vi "cursor manipulation.vi"(5 "cursor type":T1(ring), 6 "Cursor.Cursor Mode":u32, 7 "cursor position":T4(ring), 9 "graph reference in":refnum<vi>, 10 "y-array":dbl[](array[numeric]), 11 "x-array":dbl[](array[numeric])) -> (3 "reference out":refnum<vi>)   [LabVIEW 2021]
uses:
  <vilib>/Utility/miscctls.llb/LVCursorListTypeDef.ctl
panel:
  out "Cursor List Out":T2(array[cluster])
  out "Cursor List In":T3=[{"Name"="Cursor 0", "Color"=16775680, "Style"=0, "Point Style"=13, "Name Visible"=FALSE, "Allow Drag"=TRUE, "Cursor Mode"=1, "Plot"=0, "Index"=0, "Position"={"X"=99.93178733333333, "Y"=99.0278}, "X Scale"=0, "Y Scale"=0, "Watch Plots"=[], "Watch All Plots"=FALSE, "Plot Area"=0, "Label Offset"={"X"=-47.70298455485651, "Y"=-2401.3690448763255}}, {"Name"="Cursor 1", "Color"=16776960, "Style"=0, "Point Style"=13, "Name Visible"=FALSE, "Allow Drag"=TRUE, "Cursor Mode"=1, "Plot"=-1, "Index"=33, "Position"={"X"=197.3124, "Y"=196.0}, "X Scale"=0, "Y Scale"=0, "Watch Plots"=[], "Watch All Plots"=FALSE, "Plot Area"=0, "Label Offset"={"X"=24.672569516556308, "Y"=-2417.1156279151946}}]
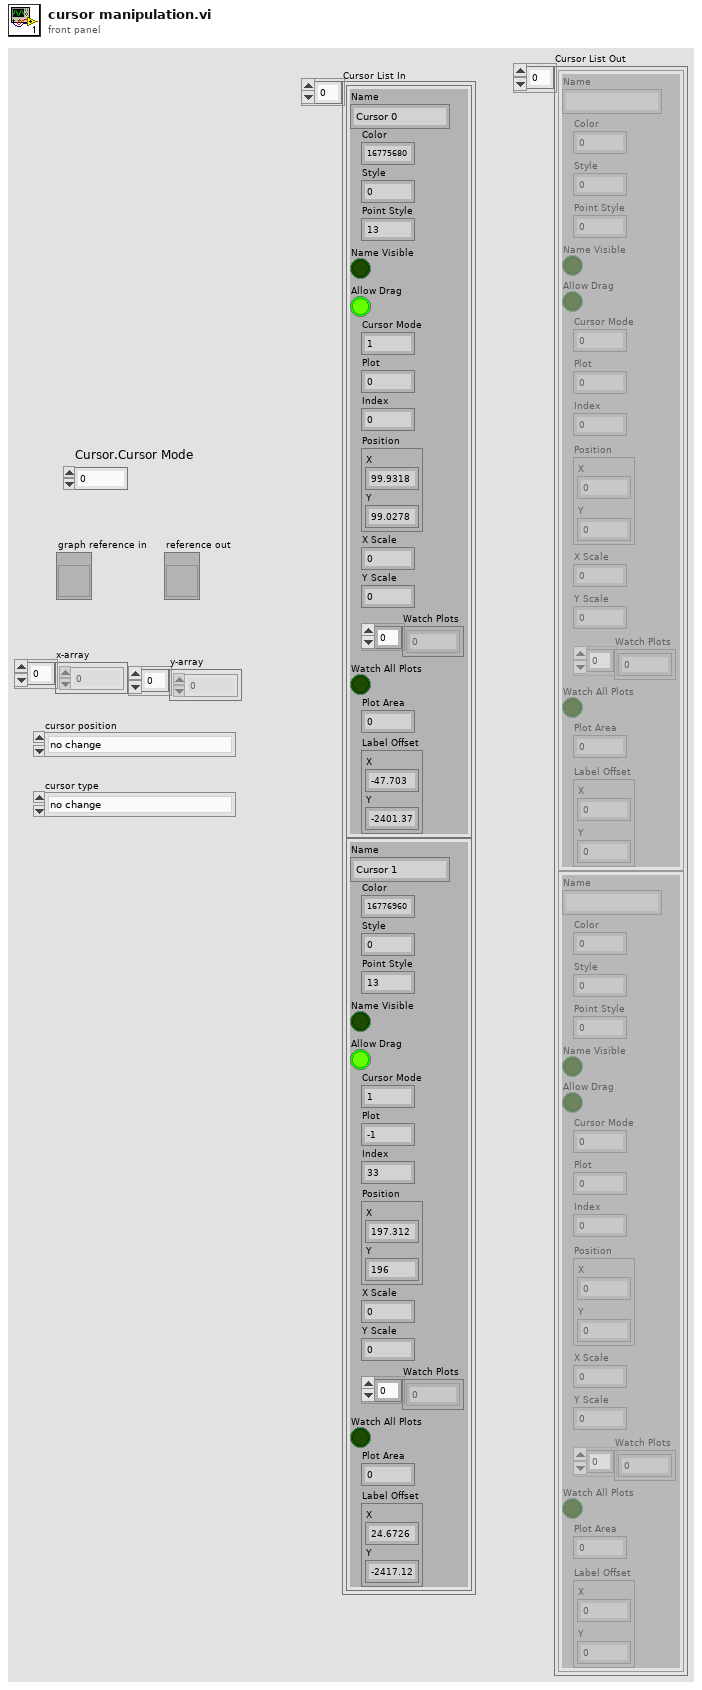
[diagram p1: front panel]
types:
  T1 = enum16{"no change", "hide cursor", "cross", "horizontal", "vertical"}
  T2 = cluster{"Name":string, "Color":u32, "Style":u8, "Point Style":u8, "Name Visible":bool, "Allow Drag":bool, "Cursor Mode":u32, "Plot":i32, "Index":i32, "Position":cluster{"X":dbl, "Y":dbl}, "X Scale":u32, "Y Scale":u32, "Watch Plots":i32[], "Watch All Plots":bool, "Plot Area":i32, "Label Offset":cluster{"X":dbl, "Y":dbl}}[]
  T3 = typedef "LVCursorListTypeDef.ctl" = cluster{"Name":string, "Color":u32, "Style":u8, "Point Style":u8, "Name Visible":bool, "Allow Drag":bool, "Cursor Mode":u32, "Plot":i32, "Index":i32, "Position":cluster{"X":dbl, "Y":dbl}, "X Scale":u32, "Y Scale":u32, "Watch Plots":i32[], "Watch All Plots":bool, "Plot Area":i32, "Label Offset":cluster{"X":dbl, "Y":dbl}}[]
  T4 = enum16{"no change", "move to data center", "move to data corner", "move to panel center", "move to panel corner"}
  T5 = cluster{"Name":string, "Color":u32, "Style":u8, "Point Style":u8, "Name Visible":bool, "Allow Drag":bool, "Cursor Mode":u32, "Plot":i32, "Index":i32, "Position":cluster{"X":dbl, "Y":dbl}, "X Scale":u32, "Y Scale":u32, "Watch Plots":i32[], "Watch All Plots":bool, "Plot Area":i32, "Label Offset":cluster{"X":dbl, "Y":dbl}}
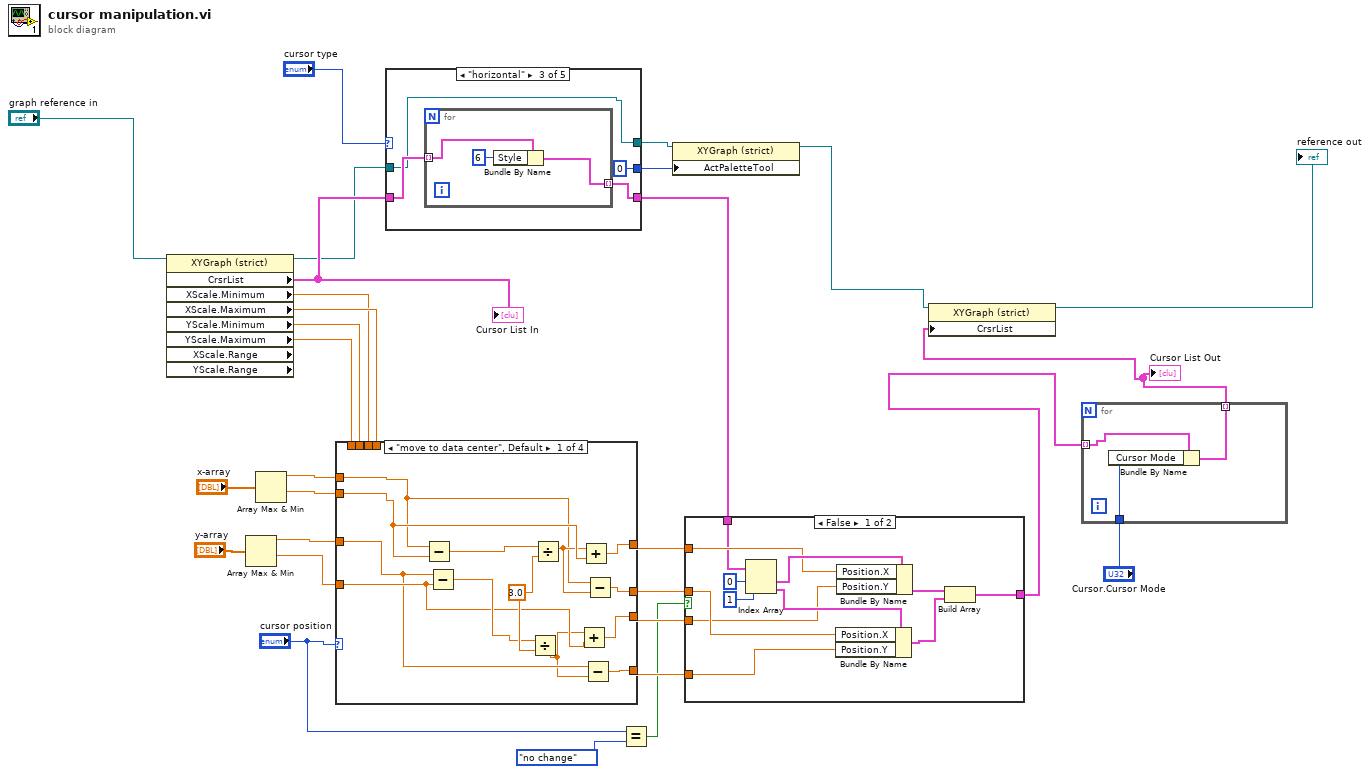
[diagram p0: block diagram]
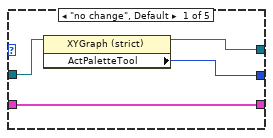
[diagram p3: hidden frame]
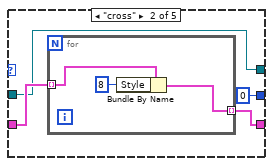
[diagram p4: hidden frame]
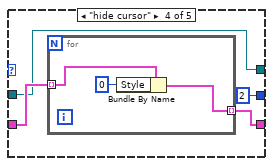
[diagram p5: hidden frame]
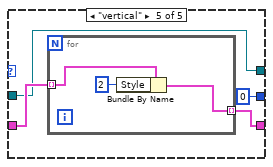
[diagram p6: hidden frame]
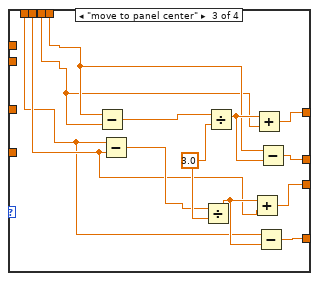
[diagram p8: hidden frame]
diagram:
  n1 = property on="Property Node" class="XYGraph (strict)" props=["CrsrList", "XScale", "Minimum", "XScale", "Maximum", "YScale", "Minimum", "YScale", "Maximum", "XScale", "Range", "YScale", "Range"](reference="graph reference in") -> (reference out=w9:refnum<vi>, "CrsrList"=w14:T3, "XScale.Minimum"=w18:dbl, "XScale.Maximum"=w19:dbl, "YScale.Minimum"=w17:dbl, "YScale.Maximum"=w16:dbl)  [unwired: 1 in, 3 out]
  "Cursor List In" <- w14
  n2 = Array Max & Min(array="y-array") -> (max value=w22:dbl, min value=w23:dbl)  [unwired: 2 out]
  n3 = Array Max & Min(array="x-array") -> (max value=w26:dbl, min value=w27:dbl)  [unwired: 2 out]
  n4 = case shown="\"move to data center\", Default" "cursor position" {
    tunnel: w27 -> [w39 w44 _ _]
    tunnel: w26 -> [w37 _ _ _]
    tunnel: [w36 w44 w52 w59] -> w25
    tunnel: [w35 w44 w51 w59] -> w24
    tunnel: w23 -> [w34 w43 _ _]
    tunnel: w22 -> [w33 _ _ _]
    tunnel: [w32 w43 w50 w58] -> w21
    tunnel: [w31 w43 w49 w58] -> w20
    tunnel: w19 -> [_ _ w48 _]
    tunnel: w18 -> [_ _ w47 w59]
    tunnel: w17 -> [_ _ w46 w58]
    tunnel: w16 -> [_ _ w45 _]
    frame "move to data center", Default {
      w41 = 3.0 ("y")
      n5 = Subtract(x=w37, y=w39) -> (x-y=w42:dbl)
      n6 = Subtract(x=w33, y=w34) -> (x-y=w40:dbl)
      n7 = Divide(x=w40, y=w41) -> (x/y=w30:dbl)
      n8 = Divide(x=w42, y=w41) -> (x/y=w38:dbl)
      n9 = Add(x=w30, y=w34) -> (x+y=w32:dbl)
      n10 = Add(x=w38, y=w39) -> (x+y=w36:dbl)
      n11 = Subtract(x=w33, y=w30) -> (x-y=w31:dbl)
      n12 = Subtract(x=w37, y=w38) -> (x-y=w35:dbl)
    }
    frame "move to data corner" {
    }
    frame "move to panel center" {
      w56 = 3.0 ("y")
      n13 = Subtract(x=w48, y=w47) -> (x-y=w57:dbl)
      n14 = Subtract(x=w45, y=w46) -> (x-y=w55:dbl)
      n15 = Divide(x=w55, y=w56) -> (x/y=w54:dbl)
      n16 = Divide(x=w57, y=w56) -> (x/y=w53:dbl)
      n17 = Add(x=w54, y=w46) -> (x+y=w50:dbl)
      n18 = Add(x=w53, y=w47) -> (x+y=w52:dbl)
      n19 = Subtract(x=w45, y=w54) -> (x-y=w49:dbl)
      n20 = Subtract(x=w48, y=w53) -> (x-y=w51:dbl)
    }
    frame "move to panel corner" {
    }
  }
  n21 = case shown="\"horizontal\"" "cursor type" {
    tunnel: w14 -> [w63 w67 w74 w81 w88]
    tunnel: [w63 w66 w73 w80 w87] -> w13
    tunnel: w9 -> [w62 w65 w72 w79 w86]
    tunnel: [w61 w65 w72 w79 w86] -> w8
    tunnel: [w60 0 ("ActPaletteTool") 0 ("ActPaletteTool") 2 ("ActPaletteTool") 0 ("ActPaletteTool")] -> w7
    frame "no change", Default {
      n22 = property class="XYGraph (strict)"(reference=w62) -> (reference out=w61:refnum<vi>, "ActPaletteTool"=w60:i32)  [unwired: 1 in, 1 out]
    }
    frame "cross" {
      n23 = for {
        tunnel: w67 -> [w70] mode=indexing
        tunnel: [w68] -> w66 mode=indexing
        n24 = Bundle By Name(cluster=w70, "Style"=u8 8) -> (w68:T5)
      }
    }
    frame "horizontal" {
      n25 = for {
        tunnel: w74 -> [w77] mode=indexing
        tunnel: [w75] -> w73 mode=indexing
        n26 = Bundle By Name(cluster=w77, "Style"=u8 6) -> (w75:T5)
      }
    }
    frame "hide cursor" {
      n27 = for {
        tunnel: w81 -> [w84] mode=indexing
        tunnel: [w82] -> w80 mode=indexing
        n28 = Bundle By Name(cluster=w84, "Style"=u8 0) -> (w82:T5)
      }
    }
    frame "vertical" {
      n29 = for {
        tunnel: w88 -> [w91] mode=indexing
        tunnel: [w89] -> w87 mode=indexing
        n30 = Bundle By Name(cluster=w91, "Style"=u8 2) -> (w89:T5)
      }
    }
  }
  n31 = Equal?(x="cursor position", y=T4."no change") -> (x = y?=w10:bool)
  n32 = property class="XYGraph (strict)"(reference=w8, "ActPaletteTool"=w7) -> (reference out=w3:refnum<vi>)  [unwired: 1 in, 1 out]
  n33 = case shown="False" w10 {
    tunnel: w25 -> [w98 _]
    tunnel: w24 -> [w97 _]
    tunnel: w21 -> [w96 _]
    tunnel: w20 -> [w95 _]
    tunnel: w13 -> [w94 w104]
    tunnel: [w92 w104] -> w4
    frame False {
      n34 = Index Array(array=w94, index #1=0 ("index"), index #2=1 ("index")) -> (element #1=w101:T5, element #2=w100:T5)
      n35 = Bundle By Name(cluster=w100, "Position.X"=w97, "Position.Y"=w95) -> (w93:T5)
      n36 = Bundle By Name(cluster=w101, "Position.X"=w98, "Position.Y"=w96) -> (w99:T5)
      n37 = Build Array(w99, w93) -> (w92:T2)
    }
    frame True {
    }
  }
  n38 = for {
    tunnel: w4 -> [w107] mode=indexing
    tunnel: "Cursor.Cursor Mode" -> [w106]
    tunnel: [w105] -> w1 mode=indexing
    n39 = Bundle By Name(cluster=w107, "Cursor Mode"=w106) -> (w105:T5)
  }
  "Cursor List Out" <- w1
  n40 = property class="XYGraph (strict)"(reference=w3, "CrsrList"=w1) -> (reference out=→"reference out":refnum<vi>)  [unwired: 1 in, 1 out]
